vi "Beam_Name_2_WaveLength.vi"(1 "Beam Name":string) -> (0 "Wavelength nm":string="488")   [LabVIEW 2011]
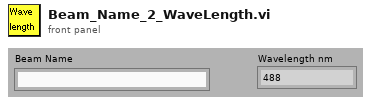
[diagram p1: front panel]
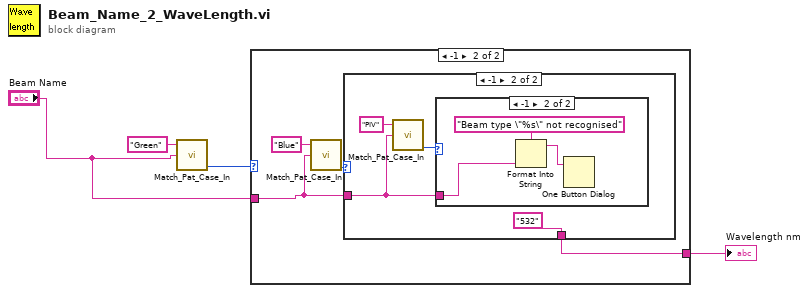
[diagram p0: block diagram]
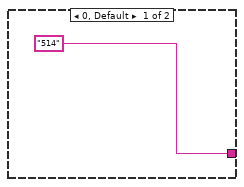
[diagram p2: hidden frame]
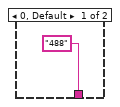
[diagram p3: hidden frame]
diagram:
  n1 = call "Match_Pat_Case_In.vi"("String to match"="Green", "String"="Beam Name") -> ("offset past match"=w3:i32)  [unwired: 1 in, 3 out]
  n2 = case shown="-1" w3 {
    tunnel: "Beam Name" -> [_ w7]
    tunnel: ["514" w6] -> w1
    frame 0, Default {
    }
    frame -1 {
      n3 = call "Match_Pat_Case_In.vi"("String to match"="Blue", "String"=w7) -> ("offset past match"=w8:i32)  [unwired: 1 in, 3 out]
      n4 = case shown="-1" w8 {
        tunnel: w7 -> [_ w11]
        tunnel: ["488" "532"] -> w6
        frame 0, Default {
        }
        frame -1 {
          n5 = call "Match_Pat_Case_In.vi"("String to match"="PIV", "String"=w11) -> ("offset past match"=w13:i32)  [unwired: 1 in, 3 out]
          n6 = case shown="-1" w13 {
            tunnel: w11 -> [_ w16]
            frame 0, Default {
            }
            frame -1 {
              n7 = Format Into String(format string="Beam type \"%s\" not recognised", w16) -> (resulting string=w15:string)  [unwired: 2 in, 1 out]
              n8 = One Button Dialog(message=w15) -> ()  [unwired: 2 out]
            }
          }
        }
      }
    }
  }
  "Wavelength nm" <- w1
